vi "CalcMultiImage.vi"() -> ()   [LabVIEW 2014]
uses:
  <userlib>/Nanonis Prog Interface V5/Nanonis Prog Interface.lvlib
panel:
  out "ETA":timestamp format="%<%H:%M\n%d/%m/%Y>T"
  out "Total time":sgl format="%<%H:%M:%S>t"
  in  "letterbox factor":sgl
  in  "# of images":sgl
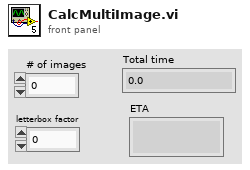
[diagram p1: front panel]
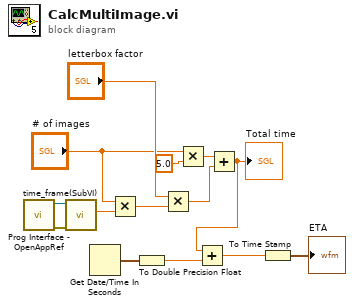
[diagram p0: block diagram]
diagram:
  n1 = call <userlib>:"Prog Interface - OpenAppRef.vi"() -> ("Error out"=w14:errorcluster, "Application reference"=w13:refnum<vi>)  [unwired: 6 in]
  n2 = call "time_frame(SubVI).vi"("error in (no error)"=w14, "Application in"=w13) -> ("Numeric"=w12:sgl)  [unwired: 7 in, 2 out]
  n3 = Get Date/Time In Seconds() -> (seconds since 1Jan1904=w5:timestamp)
  n4 = Multiply(x="# of images", y=w12) -> (x*y=w11:sgl)
  n5 = To Double Precision Float(number=w5) -> (double precision float=w4:dbl)
  n6 = Multiply(x="letterbox factor", y=w11) -> (x*y=w9:sgl)
  n7 = Multiply(x="# of images", y=sgl 5.0) -> (x*y=w8:sgl)
  n8 = Add(x=w8, y=w9) -> (x+y=w1:sgl)
  "Total time" <- w1
  n9 = Add(x=w1, y=w4) -> (x+y=w3:dbl)
  n10 = To Time Stamp(1:w3) -> (0:→"ETA":timestamp)
